vi "Write Stop checjking if OK.vi"(8 "error in (no error)":errorcluster, 10 "Stop checjking if OK":bool, 11 "Get OSF Status Msg in":refnum<class "Get OSF Status Msg.lvclass">) -> (0 "error out":errorcluster, 3 "Get OSF Status Msg out":refnum<class "Get OSF Status Msg.lvclass">)   [LabVIEW 2020, in "Get OSF Status Msg.lvclass"]
uses:
  Get OSF Status Msg.lvclass
  Get OSF Status Msg.lvclass/Get OSF Status Msg.ctl
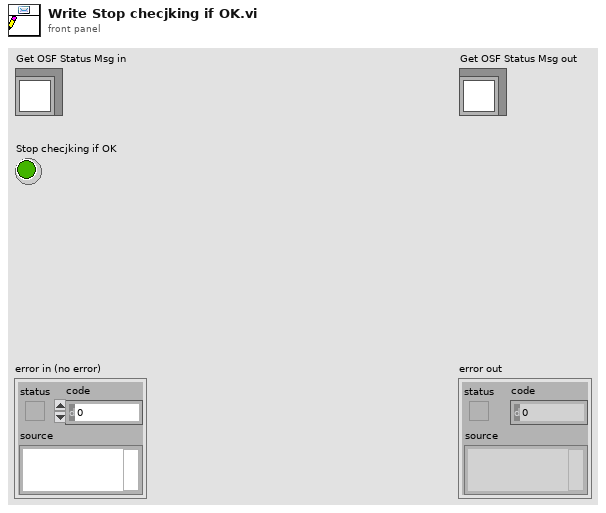
[diagram p1: front panel]
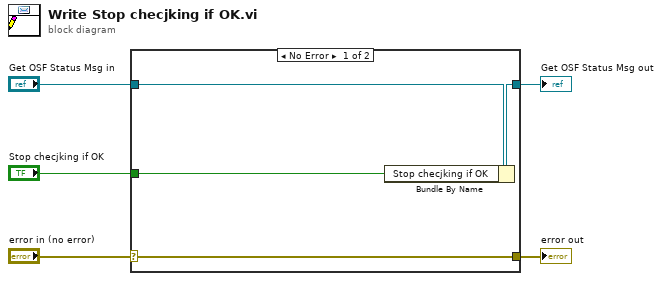
[diagram p0: block diagram]
diagram:
  n1 = case shown="No Error" "error in (no error)" {
    selector: "error in (no error)" -> [w9 w10]
    tunnel: [w9 w10] -> w4
    tunnel: [w7 w11] -> w2
    tunnel: "Get OSF Status Msg in" -> [w8 w11]
    tunnel: "Stop checjking if OK" -> [w6 _]
    frame No Error {
      n2 = Bundle By Name(cluster=w8, "Stop checjking if OK"=w6) -> (w7:refnum<class "Get OSF Status Msg.lvclass">)
    }
    frame Error {
    }
  }
  "error out" <- w4
  "Get OSF Status Msg out" <- w2
